vi "test_struct_abs_activity.vi"() -> ()   [LabVIEW 2017]
doc: "Minimal example that demonstrates functions implemented in the SorpPropLib for absorption working pairs based on the acitvity approach."
panel:
  in  "Molar volume of second component in m3/mol (Input)":dbl=-1.0
  in  "Molar volume of first component in m3/mol (Input)":dbl=-1.0
  out "Activity coefficient of first component":cluster{dbl[], dbl[]}[](graph)=[{[1000.0, 1001.0, 1002.0, 1003.0, 1004.0, 1005.0, 1006.0, 1007.0, 1008.0, 1009.0], [-1.0, -1.0, -1.0, -1.0, -1.0, -1.0, -1.0, -1.0, -1.0, -1.0]}, {[1000.0, 1001.0, 1002.0, 1003.0, 1004.0, 1005.0, 1006.0, 1007.0, 1008.0, 1009.0], [-1.0, -1.0, -1.0, -1.0, -1.0, -1.0, -1.0, -1.0, -1.0, -1.0]}]
  out "Pressure":cluster{dbl[], dbl[]}[](graph)=[{[1000.0, 1001.0, 1002.0, 1003.0, 1004.0, 1005.0, 1006.0, 1007.0, 1008.0, 1009.0], [-1.0, -1.0, -1.0, -1.0, -1.0, -1.0, -1.0, -1.0, -1.0, -1.0]}, {[1000.0, 1001.0, 1002.0, 1003.0, 1004.0, 1005.0, 1006.0, 1007.0, 1008.0, 1009.0], [-1.0, -1.0, -1.0, -1.0, -1.0, -1.0, -1.0, -1.0, -1.0, -1.0]}]
  out "Mole fraction in liquid phase":cluster{dbl[], dbl[]}[](graph)=[{[1000.0, 1001.0, 1002.0, 1003.0, 1004.0, 1005.0, 1006.0, 1007.0, 1008.0, 1009.0], [-1.0, -1.0, -1.0, -1.0, -1.0, -1.0, -1.0, -1.0, -1.0, -1.0]}, {[1000.0, 1001.0, 1002.0, 1003.0, 1004.0, 1005.0, 1006.0, 1007.0, 1008.0, 1009.0], [-1.0, -1.0, -1.0, -1.0, -1.0, -1.0, -1.0, -1.0, -1.0, -1.0]}]
  in  "WorkingPair (Input)":T1={"no_iso"=1, "no_p_sat"=1, "path_db"="D:\\Driesel\\SorpLibLocal\\labview_wrapper\\data\\json\\sorpproplib.json", "wp_as"="lubricant", "wp_st"="POE", "wp_iso"="WilsonFixedDl", "wp_rf"="R-134a", "rf_rhol"="SaturatedLiquidDensity_EoS1", "no_rhol"=1, "rf_psat"="VaporPressure_EoS1"}
  in  "Temperature in K (Input)":dbl=300.0
  in  "Pressure in Pa (Input)":dbl=1000.0
  # "Increase pressure by 5000 Pa in steps of 1 Pa."
  # "Selecting -1: Constant molar volumes stored in data base are used for calculations!"
  # "Path to database"
  # "Name of sorbent"
  # "Name of sub-type of sorbent"
  # "Name of refrigerant"
  # "Name of isotherm"
  # "ID of isotherm"
  # "Name of calculation approach for vapor pressure"
  # "ID of vapor pressure equation"
  # "Name of calculation approach for liquid density"
  # "ID of liquid density equation"
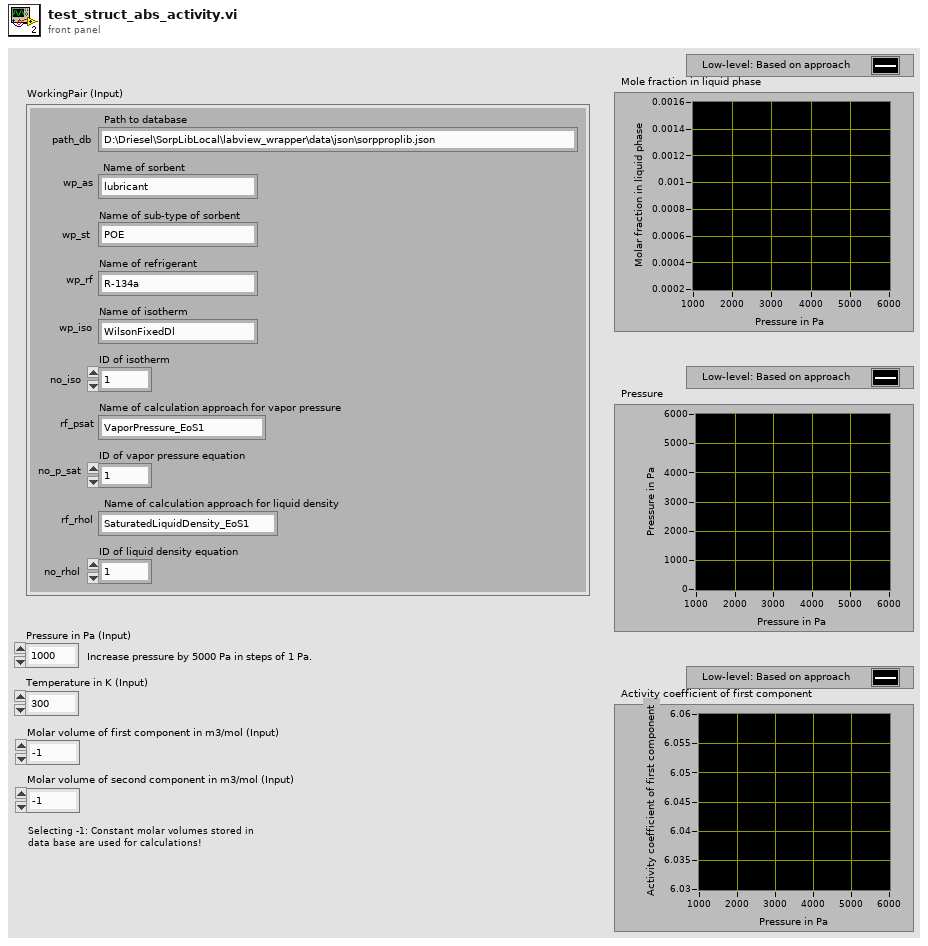
[diagram p1: front panel]
types:
  T1 = cluster{"no_iso":i32, "no_p_sat":i32, "path_db":string, "wp_as":string, "wp_st":string, "wp_iso":string, "wp_rf":string, "rf_rhol":string, "no_rhol":i32, "rf_psat":string}
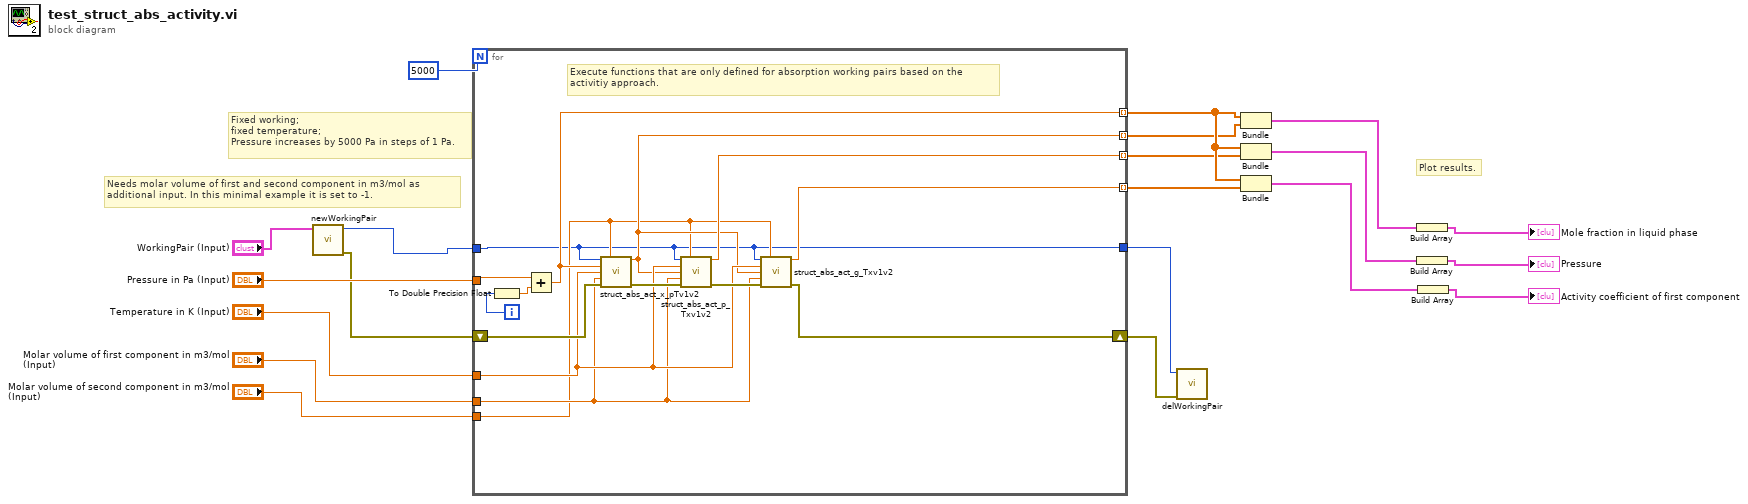
[diagram p0: block diagram]
diagram:
  # "Needs molar volume of first and second component in m3/mol as \nadditional input. In this minimal example it is set to -1."
  # "Plot results."
  # "Fixed working;\nfixed temperature;\nPressure increases by 5000 Pa in steps of 1 Pa."
  n1 = call "newWorkingPair.vi"("WorkingPair (Input)"="WorkingPair (Input)") -> ("Error (Output)"=w11:errorcluster, "workingPair"=w12:i64)  [unwired: 9 in]
  n2 = for {
    N: 5000 -> [_]
    tunnel: "Pressure in Pa (Input)" -> [w35]
    tunnel: "Temperature in K (Input)" -> [w27]
    tunnel: w12 -> [w21]
    shift-right: [w29] -> w10
    shift-left: w11 -> [w32]
    tunnel: [w28] -> w18 mode=indexing
    tunnel: [w24] -> w9 mode=indexing
    tunnel: [w26] -> w8 mode=indexing
    tunnel: [w25] -> w7 mode=indexing
    tunnel: "Molar volume of first component in m3/mol (Input)" -> [w23]
    tunnel: "Molar volume of second component in m3/mol (Input)" -> [w22]
    tunnel: [w21] -> w1
    i -> [w34]
    # "Execute functions that are only defined for absorption working pairs based on the\nactivitiy approach."
    n3 = To Double Precision Float(number=w34) -> (double precision float=w33:dbl)
    n4 = Add(x=w35, y=w33) -> (x+y=w28:dbl)
    n5 = call "struct_abs_act_x_pTv1v2.vi"("Reference working pair (Input)"=w21, "Molar volume of second component in m3/mol (Input)"=w22, "Pressure p_Pa in Pa (Input)"=w28, "Temperature in K (Input)"=w27, "Molar volume of first component in m3/mol (Input)"=w23, "Error (Input)"=w32) -> ("Mole fraction in liquid phase in mol/mol (Output)"=w24:dbl, "Error (Output)"=w31:errorcluster)  [unwired: 8 in]
    n6 = call "struct_abs_act_p_Txv1v2.vi"("Reference working pair (Input)"=w21, "Molar volume of second component in m3/mol (Input)"=w22, "Temperature in K (Input)"=w27, "Mole fraction in liquid phase in mol/mol (Input)"=w24, "Molar volume of first component in m3/mol (Input)"=w23, "Error (Input)"=w31) -> ("Pressure in Pa (Output)"=w26:dbl, "Error (Output)"=w30:errorcluster)  [unwired: 8 in]
    n7 = call "struct_abs_act_g_Txv1v2.vi"("Reference working pair (Input)"=w21, "Molar volume of second component in m3/mol (Input)"=w22, "Temperature in K (Input)"=w27, "Mole fraction in liquid phase in mol/mol (Input)"=w24, "Molar volume of first component in m3/mol (Input)"=w23, "Error (Input)"=w30) -> ("Activity coefficient of first component (Output)"=w25:dbl, "Error (Output)"=w29:errorcluster)  [unwired: 8 in]
  }
  n8 = call "delWorkingPair.vi"("Error (Input)"=w10, "workingPair"=w1) -> ()  [unwired: 9 in, 1 out]
  n9 = Bundle(w18, w9) -> (w17:cluster{dbl[], dbl[]})  [unwired: 1 in]
  n10 = Bundle(w18, w8) -> (w16:cluster{dbl[], dbl[]})  [unwired: 1 in]
  n11 = Bundle(w18, w7) -> (w15:cluster{dbl[], dbl[]})  [unwired: 1 in]
  n12 = Build Array(w17) -> (→"Mole fraction in liquid phase":cluster{dbl[], dbl[]}[])
  n13 = Build Array(w16) -> (→"Pressure":cluster{dbl[], dbl[]}[])
  n14 = Build Array(w15) -> (→"Activity coefficient of first component":cluster{dbl[], dbl[]}[])
